vi "InitConfigParams.vi"(8 "error in (no error)":errorcluster, 10 "configuration file path":path, 11 "CameraDemo in":refnum<class "CameraDemo.lvclass">) -> (0 "error out":errorcluster, 3 "CameraDemo out":refnum<class "CameraDemo.lvclass">)   [LabVIEW 2020, in "CameraI2COUSB.lvlib" / "CameraDemo.lvclass"]
uses:
  CameraDemo.lvclass
  CameraDemo.lvclass/CameraDemo.ctl
  <vilib>/Utility/config.llb/Read Key (U32).vi
  <vilib>/Utility/config.llb/Read Key (Path).vi
  <vilib>/Utility/config.llb/Read Key (String).vi
  <vilib>/Utility/config.llb/NI_LVConfig.lvlib
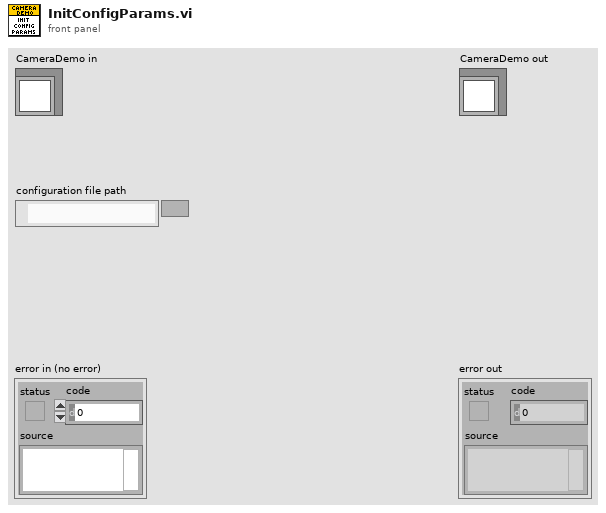
[diagram p1: front panel]
types:
  T1 = typedef "NI_LVConfig.lvlib/Config Data RefNum.ctl" = refnum<k1>
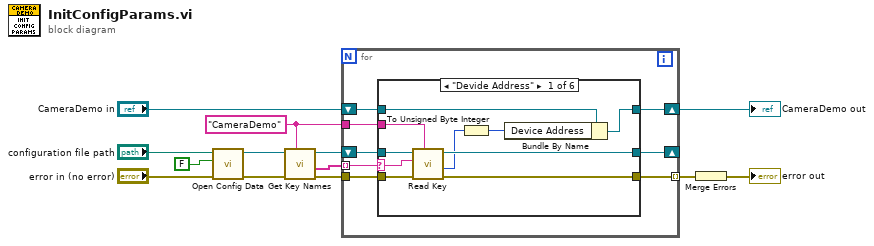
[diagram p0: block diagram]
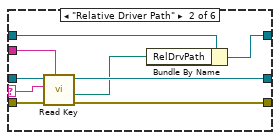
[diagram p2: hidden frame]
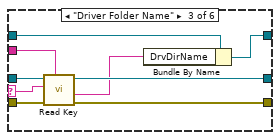
[diagram p3: hidden frame]
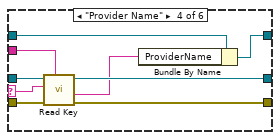
[diagram p4: hidden frame]
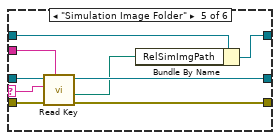
[diagram p5: hidden frame]
diagram:
  w3 = "CameraDemo" ("section")
  n1 = call <vilib>:"Open Config Data.vi"("error in (no error)"="error in (no error)", "create file if necessary (T)"=FALSE, "configuration file path"="configuration file path") -> ("error out"=w12:errorcluster, "refnum"=w11:T1)  [unwired: 6 in, 1 out]
  n2 = call <vilib>:"Get Key Names.vi"("section"=w3, "error in (no error)"=w12, "refnum"=w11) -> ("error out"=w8:errorcluster, "key names"=w10:string[], "refnum out"=w9:T1)  [unwired: 5 in, 1 out]
  n3 = for {
    tunnel: w10 -> [w21] mode=indexing
    shift-right: [w17] -> w5
    shift-left: "CameraDemo in" -> [w20]
    shift-right: [w16] -> _
    shift-left: w9 -> [w19]
    tunnel: w8 -> [w18]
    tunnel: [w15] -> w7 mode=indexing
    tunnel: w3 -> [w14]
    n4 = case shown="\"Devide Address\"" w21 {
      selector: w21 -> [w29 w38 w47 w56 w65 _]
      tunnel: w20 -> [w28 w37 w46 w55 w64 w70]
      tunnel: w19 -> [w30 w39 w48 w57 w66 w69]
      tunnel: w18 -> [w31 w40 w49 w58 w67 w68]
      tunnel: [w27 w36 w45 w54 w63 w70] -> w17
      tunnel: [w26 w35 w44 w53 w62 w69] -> w16
      tunnel: [w25 w34 w43 w52 w61 w68] -> w15
      tunnel: w14 -> [w22 w32 w41 w50 w59 _]
      frame "Devide Address" {
        n5 = call-poly <vilib>:"Read Key.vi"("section"=w22, "error in (no error)"=w31, "key"=w29, "refnum"=w30) -> ("error out"=w25:errorcluster, "value"=w23:u32, "refnum out"=w26:T1)  [unwired: 4 in, 1 out]
        n6 = To Unsigned Byte Integer(number=w23) -> (unsigned 8bit integer=w24:u8)
        n7 = Bundle By Name(cluster=w28, "Device Address"=w24) -> (w27:refnum<class "CameraDemo.lvclass">)
      }
      frame "Relative Driver Path" {
        n8 = call-poly <vilib>:"Read Key.vi"("section"=w32, "error in (no error)"=w40, "key"=w38, "refnum"=w39) -> ("error out"=w34:errorcluster, "value"=w33:path, "refnum out"=w35:T1)  [unwired: 4 in, 1 out]
        n9 = Bundle By Name(cluster=w37, "RelDrvPath"=w33) -> (w36:refnum<class "CameraDemo.lvclass">)
      }
      frame "Driver Folder Name" {
        n10 = call-poly <vilib>:"Read Key.vi"("section"=w41, "error in (no error)"=w49, "key"=w47, "refnum"=w48) -> ("error out"=w43:errorcluster, "value"=w42:string, "refnum out"=w44:T1)  [unwired: 4 in, 1 out]
        n11 = Bundle By Name(cluster=w46, "DrvDirName"=w42) -> (w45:refnum<class "CameraDemo.lvclass">)
      }
      frame "Provider Name" {
        n12 = call-poly <vilib>:"Read Key.vi"("section"=w50, "error in (no error)"=w58, "key"=w56, "refnum"=w57) -> ("error out"=w52:errorcluster, "value"=w51:string, "refnum out"=w53:T1)  [unwired: 4 in, 1 out]
        n13 = Bundle By Name(cluster=w55, "ProviderName"=w51) -> (w54:refnum<class "CameraDemo.lvclass">)
      }
      frame "Simulation Image Folder" {
        n14 = call-poly <vilib>:"Read Key.vi"("section"=w59, "error in (no error)"=w67, "key"=w65, "refnum"=w66) -> ("error out"=w61:errorcluster, "value"=w60:path, "refnum out"=w62:T1)  [unwired: 4 in, 1 out]
        n15 = Bundle By Name(cluster=w64, "RelSimImgPath"=w60) -> (w63:refnum<class "CameraDemo.lvclass">)
      }
      frame Default {
      }
    }
  }
  "CameraDemo out" <- w5
  n16 = Merge Errors(w7) -> (→"error out":errorcluster)
